vi "Build File Folder.vi"(6 "File Name":string="_Cap_Binning.csv", 8 "error in (no error)":errorcluster, 11 "TMN DC\\CAP Data Log File Path":path) -> (0 "error out":errorcluster, 2 "size (in bytes)":i64, 3 "Byte Stream File out":refnum<file>)   [LabVIEW 2017]
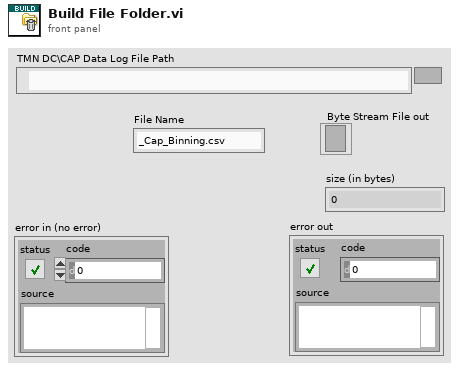
[diagram p1: front panel]
types:
  T1 = enum16{"open", "replace", "create", "open or create", "replace or create", "replace or create with confirmation"}
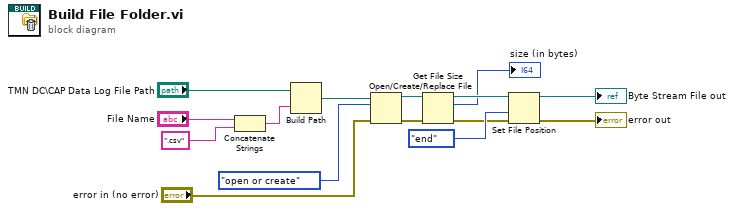
[diagram p0: block diagram]
diagram:
  n1 = Concatenate Strings("File Name", ".csv" ("string")) -> (w13:string)
  n2 = Build Path(base path="TMN DC\\CAP Data Log File Path", name or relative path=w13) -> (appended path=w4:path)
  n3 = Open/Create/Replace File(file path (use dialog)=w4, error in="error in (no error)", operation (0:open)=T1."open or create") -> (refnum out=w5:refnum<file>, error out=w3:errorcluster)  [unwired: 4 out]
  n4 = Get File Size(file=w5, error in=w3) -> (refnum out=w10:refnum<file>, size (in bytes)=→"size (in bytes)":i64, 0:w8:errorcluster)
  n5 = Set File Position(refnum=w10, from (0:start)=enum16{"start", "end", "current"}."end", error in=w8) -> (refnum out=→"Byte Stream File out":refnum<file>, error out=→"error out":errorcluster)  [unwired: 1 out]
